vi "Second Order System RT Demo.vi"() -> ()   [LabVIEW 2020]
uses:
  <vilib>/Platform/TimedLoop/XDataNode/timing_clust.ctl
  <vilib>/Platform/TimedLoop/XDataNode/nitl_modes.ctl
  <vilib>/Platform/TimedLoop/XDataNode/wakeup.ctl
  <vilib>/platform/TimedLoop/XDataNode/XDataNode.xnode
  <vilib>/Platform/TimedLoop/XDataNode/XDNodeRunTimeDep.lvlib
panel:
  out "Meter":dbl(knob) scale=0.0..2.0
  in  "Stop":bool
  out "Vertical Fill Slide":dbl(slide)=1.0000377245410232 scale=0.0..2.0
  in  "Restart":bool
  out "Waveform Chart":waveform(dbl)(graph)={"t0"=timestamp(3630901049.0798745 s since 1904-01-01), "dt"=0.01, "Y"=[1.0000377245410232]}
  in  "Damping Ratio":dbl(slide)=0.2 min=0.0 max=2.0 step=0.05 scale=0.0..2.0
  in  "Resonance Frequency [Hz]":dbl=0.5 min=0.1 max=10.0 step=0.1
  # "Second Order System Demo"
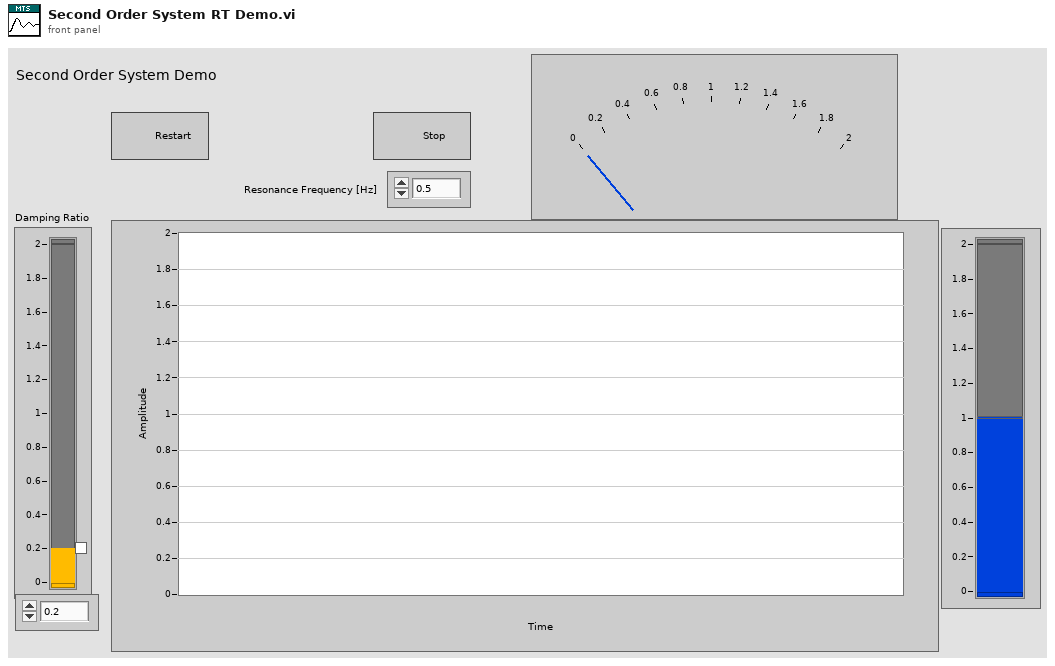
[diagram p1: front panel]
types:
  T1 = typedef "XDNodeRunTimeDep.lvlib/timing_clust.ctl" = cluster{"Expected End [f-1]":u64, "Actual End [f-1]":u64, "Finished Late? [f-1]":bool, "Expected End [i-1]":u64, "Actual End [i-1]":u64, "Finished Late? [i-1]":bool, "Expected Start [i]":u64, "Actual Start [i]":u64, "Expected Start [f]":u64, "Actual Start [f]":u64, "Source Name":string, "Structure Name":string, "Period":i64, "Deadline":i64, "Offset":i64, "Start":i64, "Priority":i32, "Timeout":i32, "Mode":T2, "Wakeup Reason":T3, "Error":errorcluster, "Source Type":string, "Secondary Source Type":string, "Global End Time":u64, "Global Start Time":u64, "Frame Duration":u64, "Iteration Duration":u64, "Assigned CPU":i32, "I/O Scan Engine Mode":u32}
  T2 = typedef "XDNodeRunTimeDep.lvlib/nitl_modes.ctl" = enum32{"No Change", "Process missed periods, maintain original phase", "Discard missed periods, maintain original phase", "Process missed periods, ignore original phase", "Discard missed periods, ignore original phase"}
  T3 = typedef "XDNodeRunTimeDep.lvlib/wakeup.ctl" = enum32{"Normal", "Aborted", "Asynchronous wakeup", "Timing source error", "Timed loop error", "Timeout"}
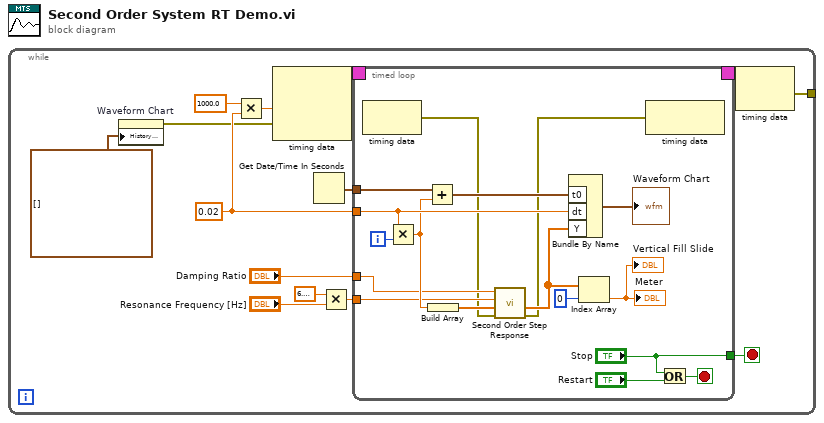
[diagram p0: block diagram]
diagram:
  n1 = while {
    tunnel: [w2] -> _
    stop <- w7 stop-if-true
    w11 = 0.02 ("dt [s]")
    n2 = property on="Waveform Chart" class="WFChart (strict)"("History Data"=waveform(dbl)[] []) -> (error out=w1:errorcluster)  [unwired: 2 in, 1 out]
    n3 = Multiply(x=1000.0 ("y"), y=w11) -> (x*y=w12:dbl)
    n4 = node-c288(w12, w1) -> (w14:T1)  [unwired: 1 in]
    n5 = Get Date/Time In Seconds() -> (seconds since 1Jan1904=w9:timestamp)
    n6 = Multiply(x=6.283185307179586, y="Resonance Frequency [Hz]") -> (x*y=w3:dbl)
    n7 = timed-loop {
      timing: w14 -> [_]
      timing-out: [_] -> w13
      tunnel: w11 -> [w28]
      tunnel: w9 -> [w27]
      tunnel: ["Stop"] -> w7
      tunnel: "Damping Ratio" -> [w19]
      tunnel: w3 -> [w18]
      i -> [w31]
      stop <- w21 stop-if-true
      n8 = node-c288() -> (w17:errorcluster)  [unwired: 1 in]
      n9 = Multiply(x=w28, y=w31) -> (x*y=w25:dbl)
      n10 = Add(x=w27, y=w25) -> (x+y=w26:timestamp)
      n11 = Build Array(w25) -> (w30:dbl[])
      n12 = call "Second Order Step Response.vi"("Error In"=w17, "Time [s]"=w30, "w0"=w18, "xi"=w19) -> ("Error Out"=w16:errorcluster, "Response"=w24:dbl[])  [unwired: 6 in]
      n13 = Bundle By Name("t0"=w26, "dt"=w28, "Y"=w24) -> (→"Waveform Chart":waveform(dbl))  [unwired: 1 in]
      n14 = Index Array(array=w24, index=0) -> (element=→"Vertical Fill Slide" →"Meter":dbl)
      n15 = node-c288(w16) -> ()  [unwired: 1 out]
      n16 = Or(x="Stop", y="Restart") -> (x .or. y?=w21:bool)
    }
    n17 = node-c288(w13) -> (w2:errorcluster)
  }
